vi "setVerticalCoupling.vi"(7 "Chn":string, 8 "error in (no error)":errorcluster, 10 "Coupling":T1, 11 "ScopeKeysight in":refnum<class "ScopeKeysight.lvclass">) -> (0 "error out":errorcluster, 3 "ScopeKeysight out":refnum<class "ScopeKeysight.lvclass">)   [LabVIEW 2023, in "ScopeKeysight.lvclass"]
doc: "<b>Author:</b> Wolfgang\n<b>Description:</b> specify the input coupling of the channel."
uses:
  ScopeKeysight.lvclass
  Data/scopeChnCoupling.ctl
  ScopeKeysight.lvclass/ScopeKeysight.ctl
  Driver/Keysight-DSQx3014T.lvlib
  sweScope.lvlib
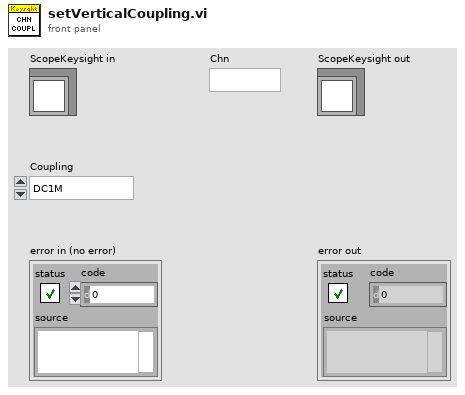
[diagram p1: front panel]
types:
  T1 = typedef "sweScope.lvlib/scopeChnCoupling.ctl" = enum16{"DC1M", "AC1M", "DC50", "GND"}
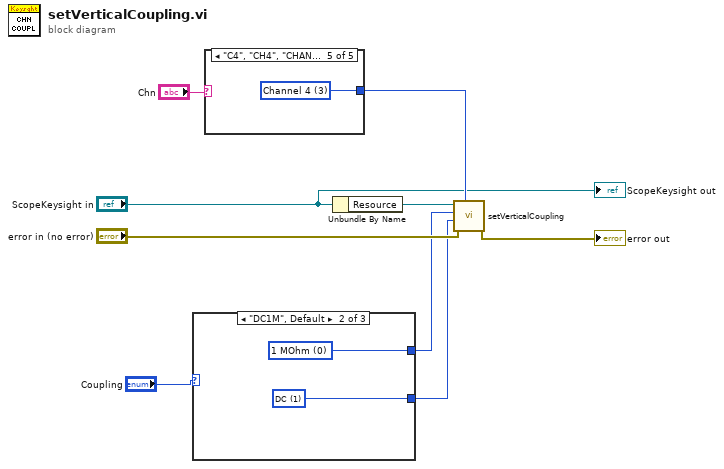
[diagram p0: block diagram]
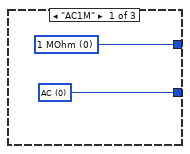
[diagram p2: hidden frame]
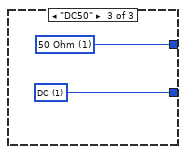
[diagram p3: hidden frame]
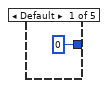
[diagram p4: hidden frame]
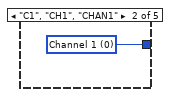
[diagram p5: hidden frame]
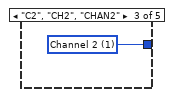
[diagram p6: hidden frame]
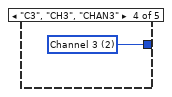
[diagram p7: hidden frame]
diagram:
  n1 = case shown="\"DC1M\", Default" "Coupling" {
    tunnel: [w11 w13 w15] -> w2
    tunnel: [w10 w12 w14] -> w1
    frame "AC1M" {
      w10 = 0 items=["AC", "DC"] ("Coupling (1: DC)")
      w11 = 0 items=["1 MOhm", "50 Ohm"] ("Impedance (0: 1 MOhm)")
    }
    frame "DC1M", Default {
      w12 = 1 items=["AC", "DC"] ("Coupling (1: DC)")
      w13 = 0 items=["1 MOhm", "50 Ohm"] ("Impedance (0: 1 MOhm)")
    }
    frame "DC50" {
      w14 = 1 items=["AC", "DC"] ("Coupling (1: DC)")
      w15 = 1 items=["1 MOhm", "50 Ohm"] ("Impedance (0: 1 MOhm)")
    }
  }
  n2 = case shown="\"C4\", \"CH4\", \"CHAN4\"" "Chn" {
    tunnel: [0 ("Channel Name (0: Channel 1)") w17 w18 w19 w20] -> w8
    frame Default {
    }
    frame "C1", "CH1", "CHAN1" {
      w17 = 0 items=["Channel 1", "Channel 2", "Channel 3", "Channel 4"] ("Channel Name (0: Channel 1)")
    }
    frame "C2", "CH2", "CHAN2" {
      w18 = 1 items=["Channel 1", "Channel 2", "Channel 3", "Channel 4"] ("Channel Name (0: Channel 1)")
    }
    frame "C3", "CH3", "CHAN3" {
      w19 = 2 items=["Channel 1", "Channel 2", "Channel 3", "Channel 4"] ("Channel Name (0: Channel 1)")
    }
    frame "C4", "CH4", "CHAN4" {
      w20 = 3 items=["Channel 1", "Channel 2", "Channel 3", "Channel 4"] ("Channel Name (0: Channel 1)")
    }
  }
  n3 = Unbundle By Name("ScopeKeysight in") -> ("Resource"=w7:refnum<visa-resource-name>)
  n4 = call "setVerticalCoupling.vi"("Channel Name (0: Channel 1)"=w8, "error in (no error)"="error in (no error)", "Coupling (1: DC)"=w1, "Impedance (0: 1 MOhm)"=w2, "VISA resource name"=w7) -> ("error out"=→"error out":errorcluster)  [unwired: 5 in, 1 out]
  "ScopeKeysight out" <- "ScopeKeysight in"
